vi "Log2txt.vi"() -> ()   [LabVIEW 2010]
panel:
  in  "number of acquisitions":i32=10 min=1 max=100
  out "data":sgl[](graph)
  in  "number of points/acquisition":i32=10
  # "Instructions:\n1. Select number of acquisitions and \n    number of points/acquisition.\n2. Run VI.\n3. When file dialog appears, select\n    file to replace or create new file.\n4. Run Read from Text File.vi to \n    read file generated with this VI."
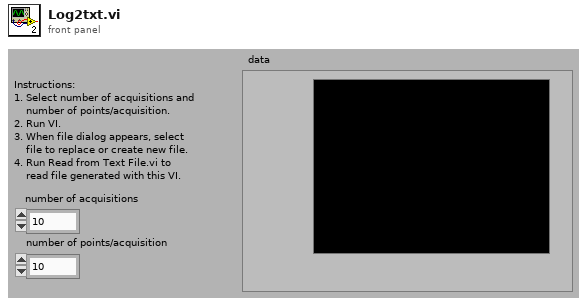
[diagram p1: front panel]
types:
  T1 = enum16{"open", "replace", "create", "open or create", "replace or create", "replace or create with confirmation"}
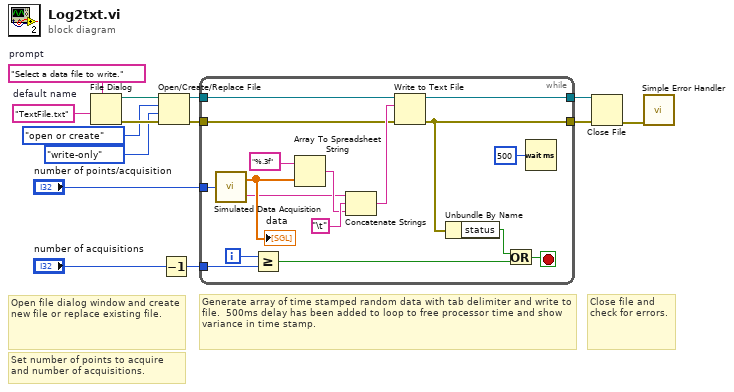
[diagram p0: block diagram]
diagram:
  w7 = "TextFile.txt"  # default name
  w6 = "Select a data file to write."  # prompt
  # "Close file and \ncheck for errors."
  # "Generate array of time stamped random data with tab delimiter and write to file.  500ms delay has been added to loop to free processor time and show variance in time stamp."
  # "Set number of points to acquire and number of acquisitions."
  # "Open file dialog window and create new file or replace existing file."
  n1 = File Dialog(7:w6, 9:w7) -> (0:w5:errorcluster, 3:w8:path)  [unwired: 1 in, 6 out]
  n2 = Open/Create/Replace File(file path (use dialog)=w8, error in=w5, operation (0:open)=T1."open or create", access (0:read/write)=enum16{"read/write", "read-only", "write-only"}."write-only") -> (refnum out=w4:refnum<file>, error out=w3:errorcluster)  [unwired: 3 out]
  n3 = Decrement(x="number of acquisitions") -> (x-1=w9:i32)
  n4 = while {
    tunnel: [w21] -> w13
    tunnel: [w20] -> w12
    tunnel: "number of points/acquisition" -> [w31]
    tunnel: w9 -> [w17]
    tunnel: w4 -> [w16]
    tunnel: w3 -> [w15]
    i -> [w26]
    stop <- w25 stop-if-true
    n5 = call "Simulated Data Acquisition.vi"("# of points"=w31) -> ("data"=w23:sgl[], "time"=w22:string)
    "data" <- w23
    n6 = Greater Or Equal?(x=w26, y=w17) -> (x >= y?=w27:bool)
    n7 = Array To Spreadsheet String(array=w23, 3:"%.3f") -> (spreadsheet string=w29:string)  [unwired: 1 out]
    n8 = Concatenate Strings(w22, "\t" ("Tab"), w29) -> (w19:string)
    n9 = Write to Text File(file (use dialog)=w16, text=w19, error in=w15) -> (refnum out=w21:refnum<file>, error out=w20:errorcluster)  [unwired: 1 in, 1 out]
    n10 = Unbundle By Name(w20) -> ("status"=w28:bool)
    n11 = Or(x=w28, y=w27) -> (x .or. y?=w25:bool)
    n12 = Wait (ms)(milliseconds to wait=u32 500 ("millisecond multiple")) -> ()  [unwired: 1 out]
  }
  n13 = Close File(refnum=w13, error in=w12) -> (error out=w11:errorcluster)  [unwired: 1 out]
  n14 = call <vilib>:"Simple Error Handler.vi"("error in (no error)"=w11) -> ()  [unwired: 1 in, 8 out]
